vi "Heizung Uebertemperatur.vi"(6 "Aktionen":T1, 8 "Fehler (Eingang)":errorcluster, 10 "Heizung Übertemperatur":bool) -> (0 "Fehler (Ausgang)":errorcluster, 2 "Heizung Übertemperatur":bool)   [LabVIEW 2020, in "Stoermeldungen.lvlib"]
uses:
  Stoermeldungen.lvlib
  Aktion Heizung Uebertemperatur.ctl
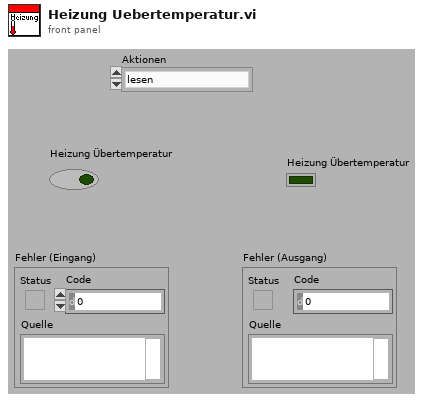
[diagram p1: front panel]
types:
  T1 = typedef "Stoermeldungen.lvlib/Aktion Heizung Uebertemperatur.ctl" = enum16{"lesen", "prüfen", "rücksetzen"}
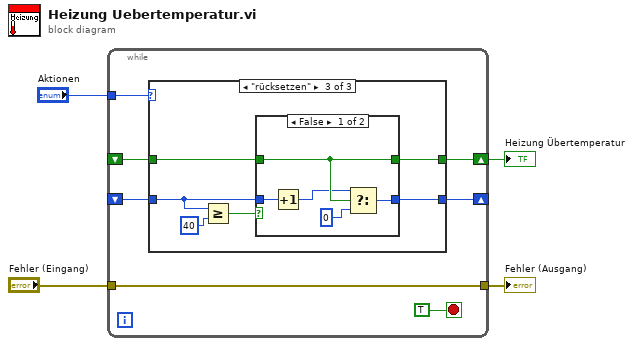
[diagram p0: block diagram]
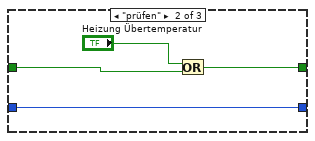
[diagram p3: hidden frame]
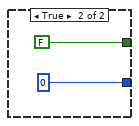
[diagram p4: hidden frame]
diagram:
  n1 = while {
    tunnel: "Aktionen" -> [w10]
    shift-right: [w9] -> w3
    shift-left: _ -> [w8]
    tunnel: [w7] -> w2
    tunnel: "Fehler (Eingang)" -> [w7]
    shift-right: [w5] -> _
    shift-left: _ -> [w6]
    stop <- TRUE stop-if-true
    n2 = case shown="\"rücksetzen\"" w10 {
      tunnel: [w13 w16 w23] -> w9
      tunnel: w8 -> [w13 w15 w19]
      tunnel: w6 -> [w12 w14 w21]
      tunnel: [w12 w14 w22] -> w5
      frame "lesen", Default {
      }
      frame "prüfen" {
        n3 = Or(x="Heizung Übertemperatur", y=w15) -> (x .or. y?=w16:bool)
      }
      frame "rücksetzen" {
        n4 = Greater Or Equal?(x=w21, y=u16 40) -> (x >= y?=w18:bool)
        n5 = case shown="False" w18 {
          tunnel: [w27 FALSE] -> w23
          tunnel: w21 -> [w28 _]
          tunnel: [w24 u16 0] -> w22
          tunnel: w19 -> [w27 _]
          frame False {
            n6 = Increment(x=w28) -> (x+1=w26:u16)
            n7 = Select(t=w26, s=w27, f=u16 0) -> (s? t:f=w24:u16)
          }
          frame True {
          }
        }
      }
    }
  }
  "Heizung Übertemperatur" <- w3
  "Fehler (Ausgang)" <- w2
